vi "Dispense X Gallons, Yoko Math Chan.vi"() -> ()   [LabVIEW 2009]
uses:
  Intellifaucet/Intellfaucet Mode.ctl
panel:
  out "Numeric":i32
  in  "y":dbl
  out "Data List":dbl[](array[numeric]) format="%.4f"
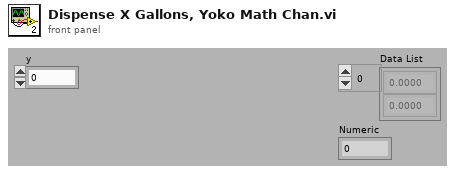
[diagram p1: front panel]
types:
  T1 = typedef "Intellfaucet Mode.ctl" = enum16{"Adjust Temp", "Adjust Flow", "Start Flow", "Stop Flow"}
  T2 = enum16{"Computation Start", "Computation stop", "Reset Computation", "Clear Computation"}[]
  T3 = typedef "Semaphore RefNum" = refnum<k1>
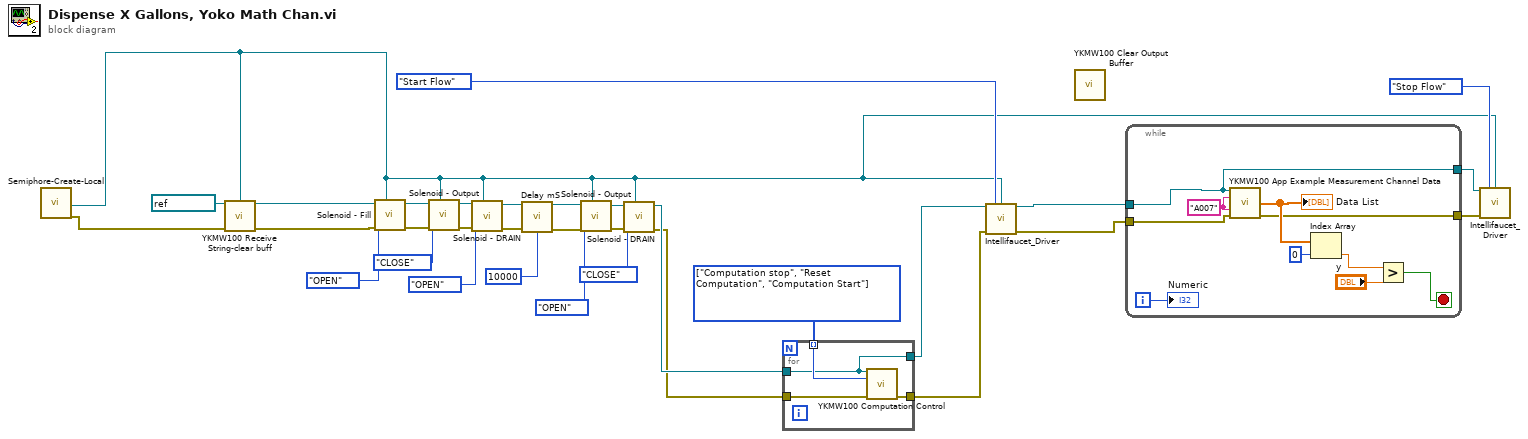
[diagram p0: block diagram]
diagram:
  w31 = T2 [enum."Computation stop", enum."Reset Computation", enum."Computation Start"] items=["Computation Start", "Computation stop", "Reset Computation", "Clear Computation"]
  n1 = call "Semiphore-Create-Local.vi"() -> ("semaphore"=w2:T3, "error out"=w5:errorcluster)  [unwired: 17 in, 1 out]
  n2 = call "YKMW100 Receive String-clear buff.vi"("VISA session"=refnum<visa-resource-name> "MW100", "Semiphore"=w2, "error in (no error)"=w5) -> ("dup VISA session"=w3:refnum<visa-resource-name>, "error out"=w4:errorcluster)  [unwired: 10 in, 1 out]
  n3 = call "Solenoid - Fill.vi"("Semiphore"=w2, "Error In"=w4, "VALVE OPEN CLOSE"=enum8{"OPEN", "CLOSE"}."OPEN", "VISA session"=w3) -> ("Error Out"=w20:errorcluster, "dup VISA session"=w25:refnum<visa-resource-name>)  [unwired: 6 in]
  n4 = call "Solenoid - Output.vi"("Semiphore"=w2, "Error In"=w20, "OPEN CLOSE"=enum8{"CLOSE", "OPEN"}."CLOSE", "VISA session"=w25) -> ("Error Out"=w19:errorcluster, "dup VISA session"=w24:refnum<visa-resource-name>)  [unwired: 6 in]
  n5 = call "Solenoid - DRAIN.vi"("Semiphore"=w2, "Error In"=w19, "VALVE OPEN CLOSE"=enum8{"OPEN", "CLOSE"}."OPEN", "VISA session"=w24) -> ("Error Out"=w18:errorcluster, "dup VISA session"=w13:refnum<visa-resource-name>)  [unwired: 6 in]
  n6 = call "Delay mS.vi"("Error In"=w18, "milliseconds to wait"=u32 10000) -> ("Error Out"=w16:errorcluster)  [unwired: 13 in]
  n7 = call "Solenoid - Output.vi"("Semiphore"=w2, "Error In"=w16, "OPEN CLOSE"=enum8{"CLOSE", "OPEN"}."OPEN", "VISA session"=w13) -> ("Error Out"=w15:errorcluster, "dup VISA session"=w14:refnum<visa-resource-name>)  [unwired: 6 in]
  n8 = call "Solenoid - DRAIN.vi"("Semiphore"=w2, "Error In"=w15, "VALVE OPEN CLOSE"=enum8{"OPEN", "CLOSE"}."CLOSE", "VISA session"=w14) -> ("Error Out"=w9:errorcluster, "dup VISA session"=w12:refnum<visa-resource-name>)  [unwired: 6 in]
  n9 = for {
    tunnel: w31 -> [w35] mode=indexing
    tunnel: w12 -> [w33]
    tunnel: [w34] -> w10
    tunnel: [w33] -> w11
    tunnel: w9 -> [w32]
    n10 = call "YKMW100 Computation Control.vi"("VISA session"=w33, "Mode"=w35, "error in (no error)"=w32) -> ("error out"=w34:errorcluster)  [unwired: 11 in, 1 out]
  }
  n11 = call "Intellifaucet_Driver.vi"("VISA session"=w11, "Mode"=Intellfaucet_Mode."Start Flow", "Semiphore"=w2, "Error In"=w10) -> ("VISA session out"=w8:refnum<visa-resource-name>, "Error Out"=w30:errorcluster)  [unwired: 10 in]
  n12 = call "YKMW100 Clear Output Buffer.vi"() -> ()  [unwired: 14 in, 2 out]
  n13 = while {
    tunnel: w30 -> [w44]
    tunnel: [w38] -> w28
    tunnel: [w37] -> w27
    tunnel: w8 -> [w37]
    i -> [w36]
    stop <- w39 stop-if-true
    w45 = "A007" ("Start Channel (001)")
    n14 = call <instrlib>:"YKMW100 App Example Measurement Channel Data.vi"("VISA session"=w37, "Start Channel (001)"=w45, "End Channel (001)"=w45, "error in (no error)"=w44) -> ("Data List"=w43:dbl[], "error out"=w38:errorcluster)  [unwired: 4 in, 6 out]
    "Data List" <- w43
    n15 = Index Array(array=w43, index=0) -> (element=w41:dbl)
    n16 = Greater?(x=w41, y="y") -> (0:w39:bool)
    "Numeric" <- w36
  }
  n17 = call "Intellifaucet_Driver.vi"("VISA session"=w27, "Mode"=Intellfaucet_Mode."Stop Flow", "Semiphore"=w2, "Error In"=w28) -> ()  [unwired: 10 in, 2 out]
